vi "Integrate & Dump.vi"(1 "Integration Time (samples)":dbl, 2 "Signal in":dbl[](array[numeric])) -> (0 "Signal out":dbl[](array[numeric]))   [LabVIEW 2009]
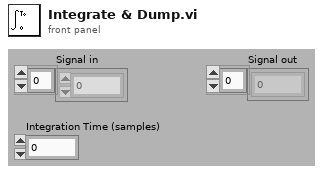
[diagram p1: front panel]
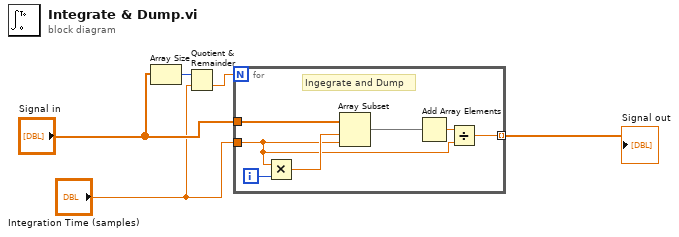
[diagram p0: block diagram]
diagram:
  n1 = Array Size(array="Signal in") -> (size(s)=w3:i32)
  n2 = Quotient & Remainder(x=w3, y="Integration Time (samples)") -> (floor(x/y)=w2:dbl)  [unwired: 1 out]
  n3 = for {
    N: w2 -> [_]
    tunnel: "Integration Time (samples)" -> [w10]
    tunnel: "Signal in" -> [w6]
    tunnel: [w9] -> w4 mode=indexing
    i -> [w12]
    # "Ingegrate and Dump"
    n4 = Multiply(x=w10, y=w12) -> (x*y=w11:dbl)
    n5 = Array Subset(array=w6, index=w11, length=w10) -> (w7:dbl[])
    n6 = Add Array Elements(numeric array=w7) -> (sum=w8:dbl)
    n7 = Divide(x=w8, y=w10) -> (x/y=w9:dbl)
  }
  "Signal out" <- w4
